vi "place in stack first row.vi"(6 "row":i32, 7 "base ang":i32, 8 "angle 2":i32, 9 "angle":i32, 10 "c2":dbl, 11 "c1":dbl) -> ()   [LabVIEW 2018]
uses:
  ARM angles.vi
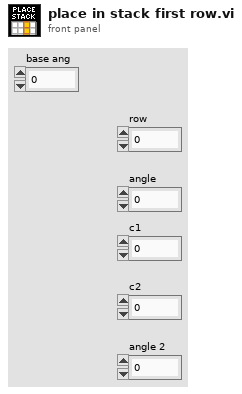
[diagram p1: front panel]
types:
  T1 = enum16{"shoulder", "elbow", "wrist", "base", "gripper"}
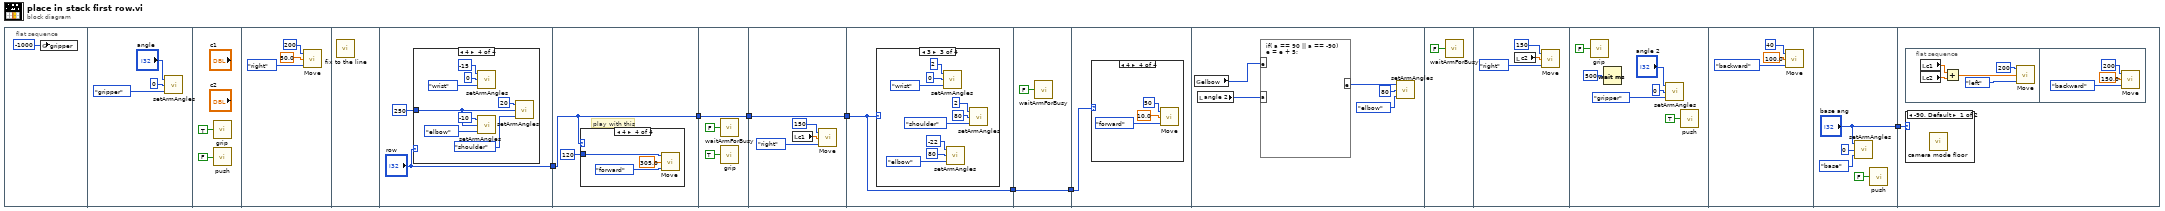
[diagram p0: block diagram]
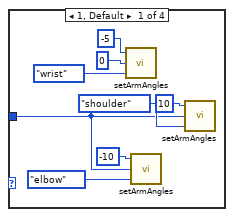
[diagram p2: hidden frame]
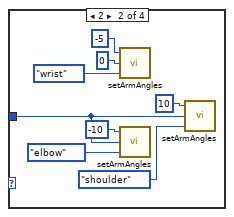
[diagram p3: hidden frame]
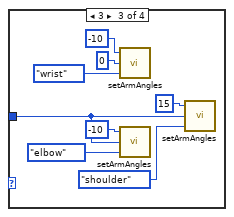
[diagram p4: hidden frame]
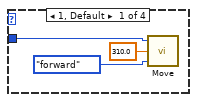
[diagram p5: hidden frame]
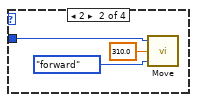
[diagram p6: hidden frame]
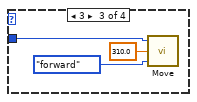
[diagram p7: hidden frame]
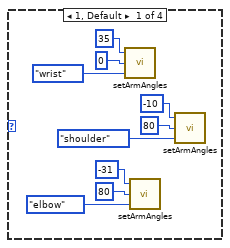
[diagram p8: hidden frame]
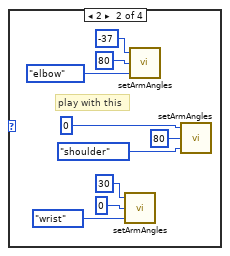
[diagram p9: hidden frame]
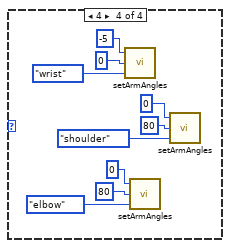
[diagram p10: hidden frame]
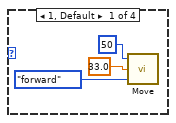
[diagram p11: hidden frame]
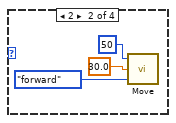
[diagram p12: hidden frame]
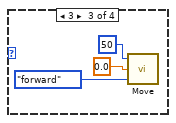
[diagram p13: hidden frame]
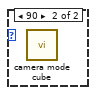
[diagram p14: hidden frame]
diagram:
  n1 = flat-sequence {
    tunnel: ["row"] -> w7
    tunnel: w7 -> [w52]
    tunnel: [w52] -> w4
    tunnel: [w65] -> w5
    tunnel: w4 -> [w65]
    tunnel: [w68] -> w6
    tunnel: w5 -> [w68]
    tunnel: w6 -> [w72]
    tunnel: [w72] -> w2
    tunnel: w2 -> [w109]
    tunnel: [w109] -> w1
    tunnel: w1 -> [w111]
    tunnel: ["base ang"] -> w3
    tunnel: w3 -> [w146]
    frame #0 {
      n2 = global write "ARM angles.vi" "gripper"(-1000 ("gripper")) -> ()
    }
    frame #1 {
      n3 = call "setArmAngles.vi"("Enum"=T1."gripper", "speed"=0, "angle"="angle") -> ()  [unwired: 1 in]
    }
    frame #2 {
      n4 = call "grip.vi"("grip"=TRUE) -> ()
      n5 = call "push.vi"("push"=FALSE) -> ()
    }
    frame #3 {
      n6 = call "Move.vi"("Enum"=enum16{"forward", "backward", "left", "right"}."right", "distance"=50.0, "speed"=200) -> ()  [unwired: 1 in]
    }
    frame #4 {
      n7 = call "fix to the line.vi"() -> ()  [unwired: 12 in]
    }
    frame #5 {
      n8 = case shown="4" "row" {
        tunnel: 250 ("speed") -> [w19 w27 w35 w43]
        frame 1, Default {
          n9 = call "setArmAngles.vi"("Enum"=T1."wrist", "speed"=0, "angle"=-5) -> ()  [unwired: 1 in]
          n10 = call "setArmAngles.vi"("Enum"=T1."elbow", "speed"=w19, "angle"=-10) -> ()  [unwired: 1 in]
          n11 = call "setArmAngles.vi"("Enum"=T1."shoulder", "speed"=w19, "angle"=10) -> ()  [unwired: 1 in]
        }
        frame 2 {
          n12 = call "setArmAngles.vi"("Enum"=T1."wrist", "speed"=0, "angle"=-5) -> ()  [unwired: 1 in]
          n13 = call "setArmAngles.vi"("Enum"=T1."elbow", "speed"=w27, "angle"=-10) -> ()  [unwired: 1 in]
          n14 = call "setArmAngles.vi"("Enum"=T1."shoulder", "speed"=w27, "angle"=10) -> ()  [unwired: 1 in]
        }
        frame 3 {
          n15 = call "setArmAngles.vi"("Enum"=T1."wrist", "speed"=0, "angle"=-10) -> ()  [unwired: 1 in]
          n16 = call "setArmAngles.vi"("Enum"=T1."elbow", "speed"=w35, "angle"=-10) -> ()  [unwired: 1 in]
          n17 = call "setArmAngles.vi"("Enum"=T1."shoulder", "speed"=w35, "angle"=15) -> ()  [unwired: 1 in]
        }
        frame 4 {
          n18 = call "setArmAngles.vi"("Enum"=T1."wrist", "speed"=0, "angle"=-15) -> ()  [unwired: 1 in]
          n19 = call "setArmAngles.vi"("Enum"=T1."elbow", "speed"=w43, "angle"=-10) -> ()  [unwired: 1 in]
          n20 = call "setArmAngles.vi"("Enum"=T1."shoulder", "speed"=w43, "angle"=20) -> ()  [unwired: 1 in]
        }
      }
    }
    frame #6 {
      # "play with this"
      n21 = case shown="4" w52 {
        tunnel: 120 ("speed") -> [w53 w56 w59 w62]
        frame 1, Default {
          n22 = call "Move.vi"("Enum"=enum16{"forward", "backward", "left", "right"}."forward", "distance"=310.0, "speed"=w53) -> ()  [unwired: 1 in]
        }
        frame 2 {
          n23 = call "Move.vi"("Enum"=enum16{"forward", "backward", "left", "right"}."forward", "distance"=310.0, "speed"=w56) -> ()  [unwired: 1 in]
        }
        frame 3 {
          n24 = call "Move.vi"("Enum"=enum16{"forward", "backward", "left", "right"}."forward", "distance"=310.0, "speed"=w59) -> ()  [unwired: 1 in]
        }
        frame 4 {
          n25 = call "Move.vi"("Enum"=enum16{"forward", "backward", "left", "right"}."forward", "distance"=305.0, "speed"=w62) -> ()  [unwired: 1 in]
        }
      }
    }
    frame #7 {
      n26 = call "waitArmForBusy.vi"("base"=FALSE) -> ()
      n27 = call "grip.vi"("grip"=TRUE) -> ()
    }
    frame #8 {
      n28 = local read "c1"() -> (w69:dbl)
      n29 = call "Move.vi"("Enum"=enum16{"forward", "backward", "left", "right"}."right", "distance"=w69, "speed"=150) -> ()  [unwired: 1 in]
    }
    frame #9 {
      n30 = case shown="3" w72 {
        frame 1, Default {
          n31 = call "setArmAngles.vi"("Enum"=T1."wrist", "speed"=0, "angle"=35) -> ()  [unwired: 1 in]
          n32 = call "setArmAngles.vi"("Enum"=T1."elbow", "speed"=80, "angle"=-31) -> ()  [unwired: 1 in]
          n33 = call "setArmAngles.vi"("Enum"=T1."shoulder", "speed"=80, "angle"=-10) -> ()  [unwired: 1 in]
        }
        frame 2 {
          # "play with this"
          n34 = call "setArmAngles.vi"("Enum"=T1."wrist", "speed"=0, "angle"=30) -> ()  [unwired: 1 in]
          n35 = call "setArmAngles.vi"("Enum"=T1."elbow", "speed"=80, "angle"=-37) -> ()  [unwired: 1 in]
          n36 = call "setArmAngles.vi"("Enum"=T1."shoulder", "speed"=80, "angle"=0) -> ()  [unwired: 1 in]
        }
        frame 3 {
          n37 = call "setArmAngles.vi"("Enum"=T1."wrist", "speed"=0, "angle"=2) -> ()  [unwired: 1 in]
          n38 = call "setArmAngles.vi"("Enum"=T1."elbow", "speed"=80, "angle"=-22) -> ()  [unwired: 1 in]
          n39 = call "setArmAngles.vi"("Enum"=T1."shoulder", "speed"=80, "angle"=2) -> ()  [unwired: 1 in]
        }
        frame 4 {
          n40 = call "setArmAngles.vi"("Enum"=T1."wrist", "speed"=0, "angle"=-5) -> ()  [unwired: 1 in]
          n41 = call "setArmAngles.vi"("Enum"=T1."elbow", "speed"=80, "angle"=0) -> ()  [unwired: 1 in]
          n42 = call "setArmAngles.vi"("Enum"=T1."shoulder", "speed"=80, "angle"=0) -> ()  [unwired: 1 in]
        }
      }
    }
    frame #10 {
      n43 = call "waitArmForBusy.vi"("base"=FALSE) -> ()
    }
    frame #11 {
      n44 = case shown="4" w111 {
        frame 1, Default {
          n45 = call "Move.vi"("Enum"=enum16{"forward", "backward", "left", "right"}."forward", "distance"=33.0, "speed"=50) -> ()  [unwired: 1 in]
        }
        frame 2 {
          n46 = call "Move.vi"("Enum"=enum16{"forward", "backward", "left", "right"}."forward", "distance"=30.0, "speed"=50) -> ()  [unwired: 1 in]
        }
        frame 3 {
          n47 = call "Move.vi"("Enum"=enum16{"forward", "backward", "left", "right"}."forward", "distance"=0.0, "speed"=50) -> ()  [unwired: 1 in]
        }
        frame 4 {
          n48 = call "Move.vi"("Enum"=enum16{"forward", "backward", "left", "right"}."forward", "distance"=10.0, "speed"=50) -> ()  [unwired: 1 in]
        }
      }
    }
    frame #12 {
      n49 = global read "ARM angles.vi" "elbow"() -> (w128:i32)
      n50 = local read "angle 2"() -> (w127:i32)
      n51 = formula code="if( a == 90 || a == -90)\ne = e + 5;"("e"=w128, "a"=w127) -> ("e"=w124:i32)
      n52 = call "setArmAngles.vi"("Enum"=T1."elbow", "speed"=80, "angle"=w124) -> ()  [unwired: 1 in]
    }
    frame #13 {
      n53 = call "waitArmForBusy.vi"("base"=FALSE) -> ()
    }
    frame #14 {
      n54 = local read "c2"() -> (w130:dbl)
      n55 = call "Move.vi"("Enum"=enum16{"forward", "backward", "left", "right"}."right", "distance"=w130, "speed"=150) -> ()  [unwired: 1 in]
    }
    frame #15 {
      n56 = call "grip.vi"("grip"=FALSE) -> ()
      n57 = Wait (ms)(milliseconds to wait=u32 500) -> ()  [unwired: 1 out]
      n58 = call "setArmAngles.vi"("Enum"=T1."gripper", "speed"=0, "angle"="angle 2") -> ()  [unwired: 1 in]
      n59 = call "push.vi"("push"=TRUE) -> ()
    }
    frame #16 {
      n60 = call "Move.vi"("Enum"=enum16{"forward", "backward", "left", "right"}."backward", "distance"=100.0, "speed"=40) -> ()  [unwired: 1 in]
    }
    frame #17 {
      n61 = call "setArmAngles.vi"("Enum"=T1."base", "speed"=0, "angle"="base ang") -> ()  [unwired: 1 in]
      n62 = call "push.vi"("push"=FALSE) -> ()
    }
    frame #18 {
      n63 = flat-sequence {
        frame #0 {
          n64 = local read "c1"() -> (w149:dbl)
          n65 = local read "c2"() -> (w148:dbl)
          n66 = Add(x=w149, y=w148) -> (x+y=w147:dbl)
          n67 = call "Move.vi"("Enum"=enum16{"forward", "backward", "left", "right"}."left", "distance"=w147, "speed"=200) -> ()  [unwired: 1 in]
        }
        frame #1 {
          n68 = call "Move.vi"("Enum"=enum16{"forward", "backward", "left", "right"}."backward", "distance"=150.0, "speed"=200) -> ()  [unwired: 1 in]
        }
      }
      n69 = case shown="-90, Default" w146 {
        frame -90, Default {
          n70 = call "camera mode floor.vi"() -> ()  [unwired: 12 in]
        }
        frame 90 {
          n71 = call "camera mode cube.vi"() -> ()  [unwired: 12 in]
        }
      }
    }
  }
